vi "IndexDir.vi"(4 "Tipo":enum16{"Simple", "Zig-Zag", "Retorno"}(ring), 6 "Barrido X":bool, 8 "j":i32, 9 "i":i32, 10 "Array Y":dbl[](array[numeric]), 11 "Array X":dbl[](array[numeric])) -> (0 "iY":i32, 1 "vY":dbl, 2 "iX":i32, 3 "vX":dbl)   [LabVIEW 2018]
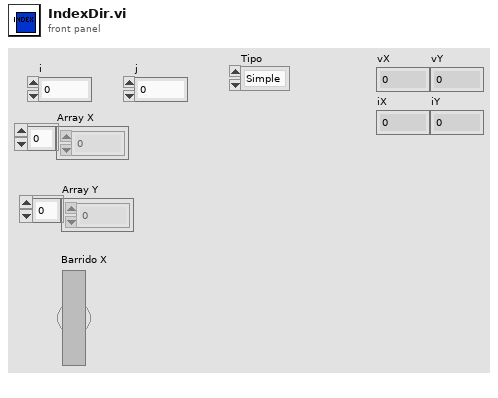
[diagram p1: front panel]
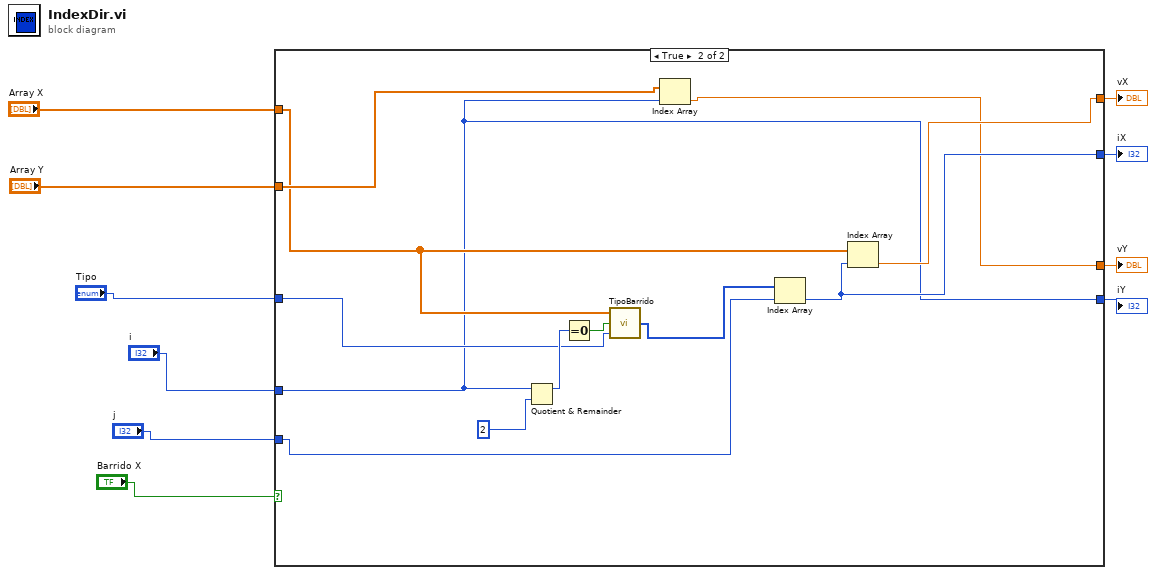
[diagram p0: block diagram]
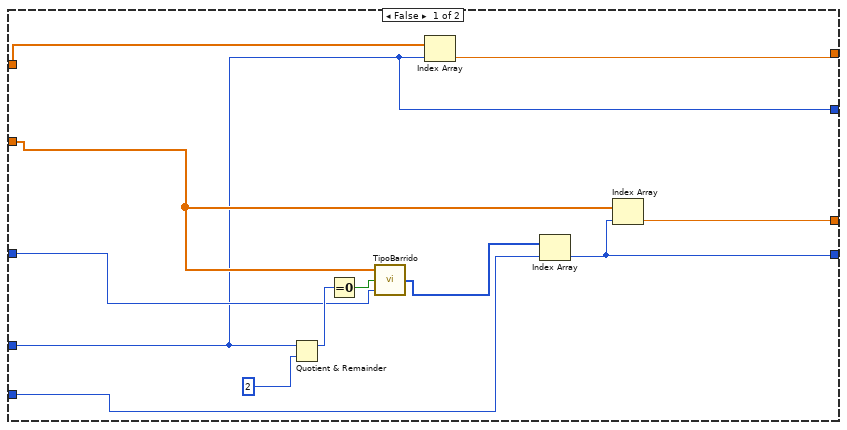
[diagram p2: hidden frame]
diagram:
  n1 = case shown="True" "Barrido X" {
    tunnel: "Array X" -> [w13 w29]
    tunnel: "Array Y" -> [w18 w30]
    tunnel: "Tipo" -> [w19 w28]
    tunnel: "i" -> [w11 w23]
    tunnel: "j" -> [w16 w27]
    tunnel: [w15 w23] -> w1
    tunnel: [w14 w24] -> w2
    tunnel: [w12 w26] -> w4
    tunnel: [w11 w25] -> w3
    frame False {
      n2 = Quotient & Remainder(x=w11, y=2) -> (x-y*floor(x/y)=w20:i32)  [unwired: 1 out]
      n3 = Equal To 0?(x=w20) -> (x = 0?=w22:bool)
      n4 = call "TipoBarrido.vi"("Tipo"=w19, "Par"=w22, "Array Y"=w18) -> ("Arr Pos"=w17:i32[])  [unwired: 1 in]
      n5 = Index Array(array=w13, index=w11) -> (element=w12:dbl)
      n6 = Index Array(array=w17, index=w16) -> (element=w15:i32)
      n7 = Index Array(array=w18, index=w15) -> (element=w14:dbl)
    }
    frame True {
      n8 = Quotient & Remainder(x=w23, y=2) -> (x-y*floor(x/y)=w32:i32)  [unwired: 1 out]
      n9 = Equal To 0?(x=w32) -> (x = 0?=w34:bool)
      n10 = call "TipoBarrido.vi"("Tipo"=w28, "Par"=w34, "Array Y"=w29) -> ("Arr Pos"=w31:i32[])  [unwired: 1 in]
      n11 = Index Array(array=w30, index=w23) -> (element=w24:dbl)
      n12 = Index Array(array=w31, index=w27) -> (element=w25:i32)
      n13 = Index Array(array=w29, index=w25) -> (element=w26:dbl)
    }
  }
  "vX" <- w4
  "iX" <- w3
  "vY" <- w2
  "iY" <- w1
